vi "Read X.vi"(8 "error in":errorcluster, 11 "PVector in":refnum<class "PVector.lvclass">) -> (0 "error out":errorcluster, 2 "X":dbl, 3 "PVector out":refnum<class "PVector.lvclass">)   [LabVIEW 2016, in "PVector.lvclass"]
uses:
  PVector.lvclass
  PVector.lvclass/PVector.ctl
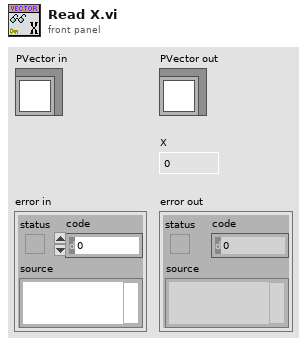
[diagram p1: front panel]
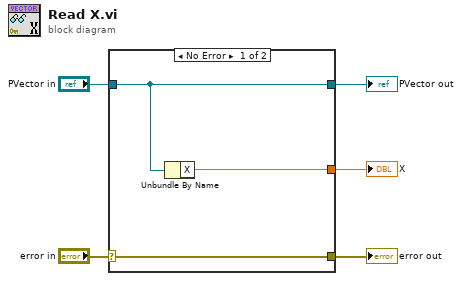
[diagram p0: block diagram]
diagram:
  n1 = case shown="No Error" "error in" {
    selector: "error in" -> [w8 w9]
    tunnel: [w8 w9] -> w4
    tunnel: [w7 w10] -> w2
    tunnel: "PVector in" -> [w7 w10]
    tunnel: [w6 _] -> w1
    frame No Error {
      n2 = Unbundle By Name(w7) -> ("X"=w6:dbl)
    }
    frame Error {
    }
  }
  "error out" <- w4
  "PVector out" <- w2
  "X" <- w1
